vi "Update PSU.vi"(4 "Error in (no error)":errorcluster, 6 "PSU Status In":T1 {"Trip Current" format="%.3f"; "Trip Field" format="%.4f"; "Voltage" format="%.2f"; "Field Constant" format="%.6f"; "MID Setpoint (T)" format="%.4f"; "MID Setpoint (A)" format="%.3f"; "MAX Setpoint (T)" format="%.4f"; "MAX Setpoint (A)" format="%.3f"; "Heater Voltage" format="%.2f"; "V Limit (V)" format="%.2f"; "Ramp Rate (A/s)" format="%.3f"; "Output (A)" format="%.3f"; "Output (T)" format="%.4f"; "Persistent Current" format="%.3f"; "Persistent Field" format="%.4f"}, 7 "VISA Resource Name In":refnum<visa-resource-name>) -> (0 "Output err":errorcluster, 1 "Ramp state err":errorcluster, 2 "Sign err":errorcluster, 3 "PSU Status Out":T1 {"Trip Current" format="%.3f"; "Trip Field" format="%.4f"; "Voltage" format="%.2f"; "Field Constant" format="%.6f"; "MID Setpoint (T)" format="%.4f"; "MID Setpoint (A)" format="%.3f"; "MAX Setpoint (T)" format="%.4f"; "MAX Setpoint (A)" format="%.3f"; "Heater Voltage" format="%.2f"; "V Limit (V)" format="%.2f"; "Ramp Rate (A/s)" format="%.3f"; "Output (A)" format="%.3f"; "Output (T)" format="%.4f"; "Persistent Current" format="%.3f"; "Persistent Field" format="%.4f"})   [LabVIEW 2022 SP3, in "Magnet module.lvlib"]
doc: "Updates actual output current and ramp status of PSU"
uses:
  Magnet module.lvlib
  <instrlib>/SMS 120/Public/PSU Status.ctl
  <instrlib>/SMS 120/Cryogenic Ltd SMSXXX.lvlib
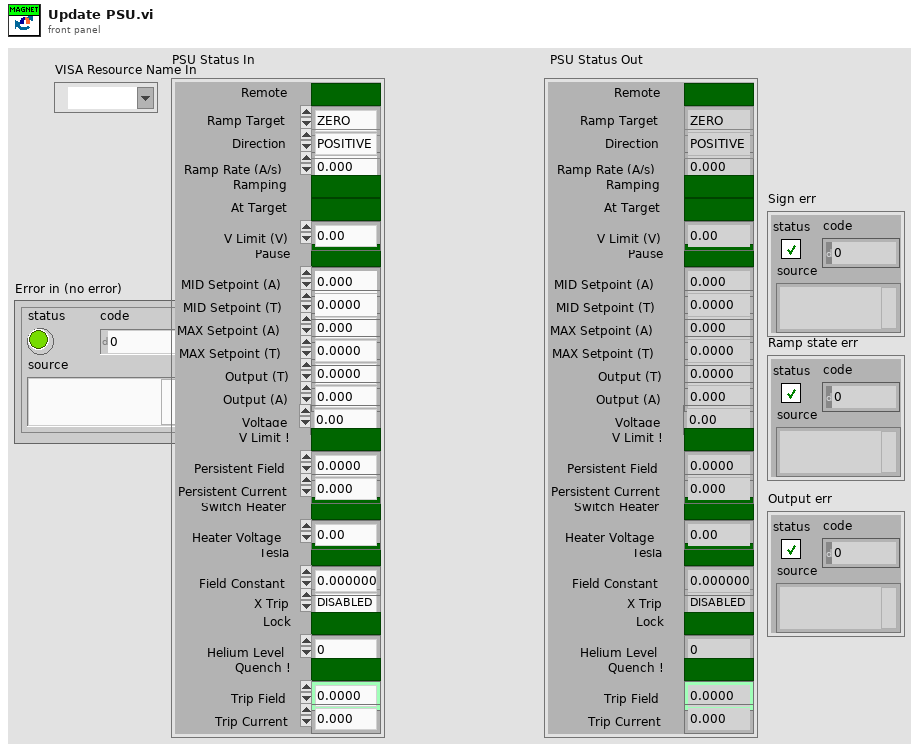
[diagram p1: front panel]
types:
  T1 = typedef "Cryogenic Ltd SMSXXX.lvlib/PSU Status.ctl" = cluster{"Ramp Target":enum16{"ZERO", "MID", "MAX"}, "Pause":bool, "Switch Heater":bool, "Persistent Field":dbl, "Persistent Current":dbl, "Tesla":bool, "Output (T)":dbl, "Output (A)":dbl, "X Trip":enum16{"DISABLED", "ENABLED", "ACTIVE"}, "Ramp Rate (A/s)":dbl, "V Limit (V)":dbl, "Heater Voltage":dbl, "MAX Setpoint (A)":dbl, "MAX Setpoint (T)":dbl, "MID Setpoint (A)":dbl, "MID Setpoint (T)":dbl, "Lock":bool, "Field Constant":dbl, "Remote":bool, "Direction":enum16{"POSITIVE", "NEGATIVE", "OPEN", "UNIPOLAR"}, "Helium Level":u16, "Quench !":bool, "Voltage":dbl, "V Limit !":bool, "Ramping":bool, "At Target":bool, "Trip Field":dbl, "Trip Current":dbl}
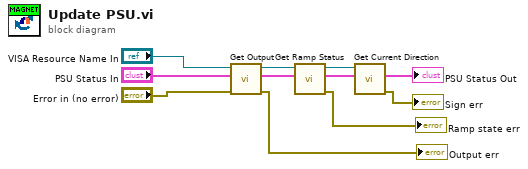
[diagram p0: block diagram]
diagram:
  n1 = call <instrlib>:"Get Output.vi"("Error in (no error)"="Error in (no error)", "PSU Status In"="PSU Status In", "VISA Resource Name In"="VISA Resource Name In") -> ("Error out"=→"Output err":errorcluster, "PSU Status Out"=w11:T1, "VISA Resource Name Out"=w10:refnum<visa-resource-name>)  [unwired: 3 in, 3 out]
  n2 = call <instrlib>:"Get Ramp Status.vi"("PSU Status In"=w11, "VISA Resource Name In"=w10) -> ("Error out"=→"Ramp state err":errorcluster, "PSU Status Out"=w5:T1, "VISA Resource Name Out"=w6:refnum<visa-resource-name>)  [unwired: 6 in, 1 out]
  n3 = call <instrlib>:"Get Current Direction.vi"("PSU Status In"=w5, "VISA Resource Name In"=w6) -> ("Error out"=→"Sign err":errorcluster, "PSU Status Out"=→"PSU Status Out":T1)  [unwired: 5 in, 3 out]
